vi "trimspace non-reentrant vs reentrant vs inline vs no-subvi.vi"() -> ()   [LabVIEW 2020]
panel:
  out "inside 4":i32
  out "[\\t\\n\\r\\s] 3":string
  out "outside 4":i32
  out "inside 3":i32
  out "[\\t\\n\\r\\s] 2":string
  out "outside 3":i32
  out "[\\t\\n\\r\\s]":string
  out "[\\t\\s]":string
  out "inside 2":i32
  out "outside 2":i32
  out "inside":i32
  out "outside":i32
  out "unit (ms)":dbl[][](graph)
  # "non-reentrant"
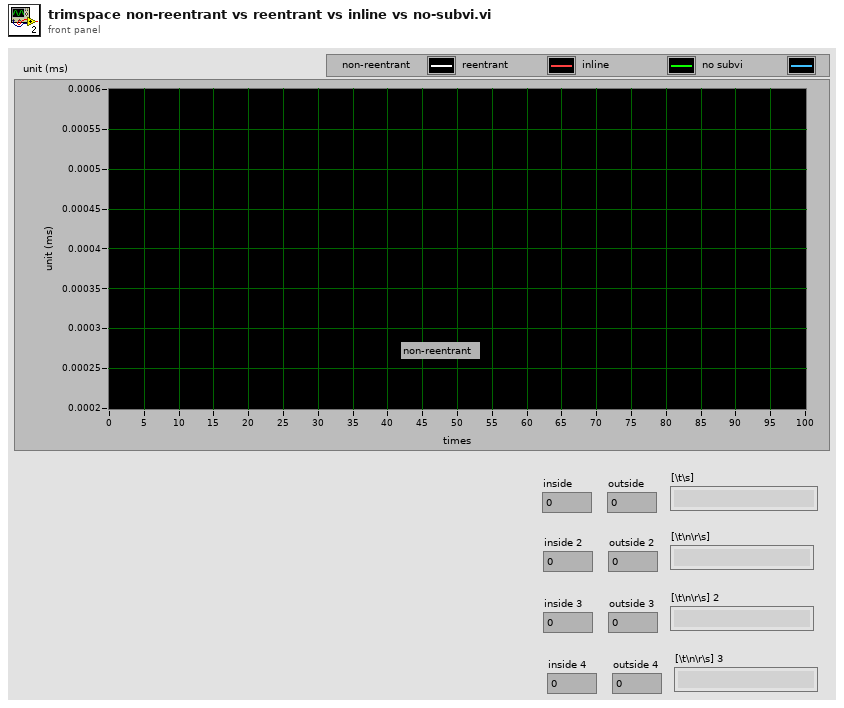
[diagram p1: front panel]
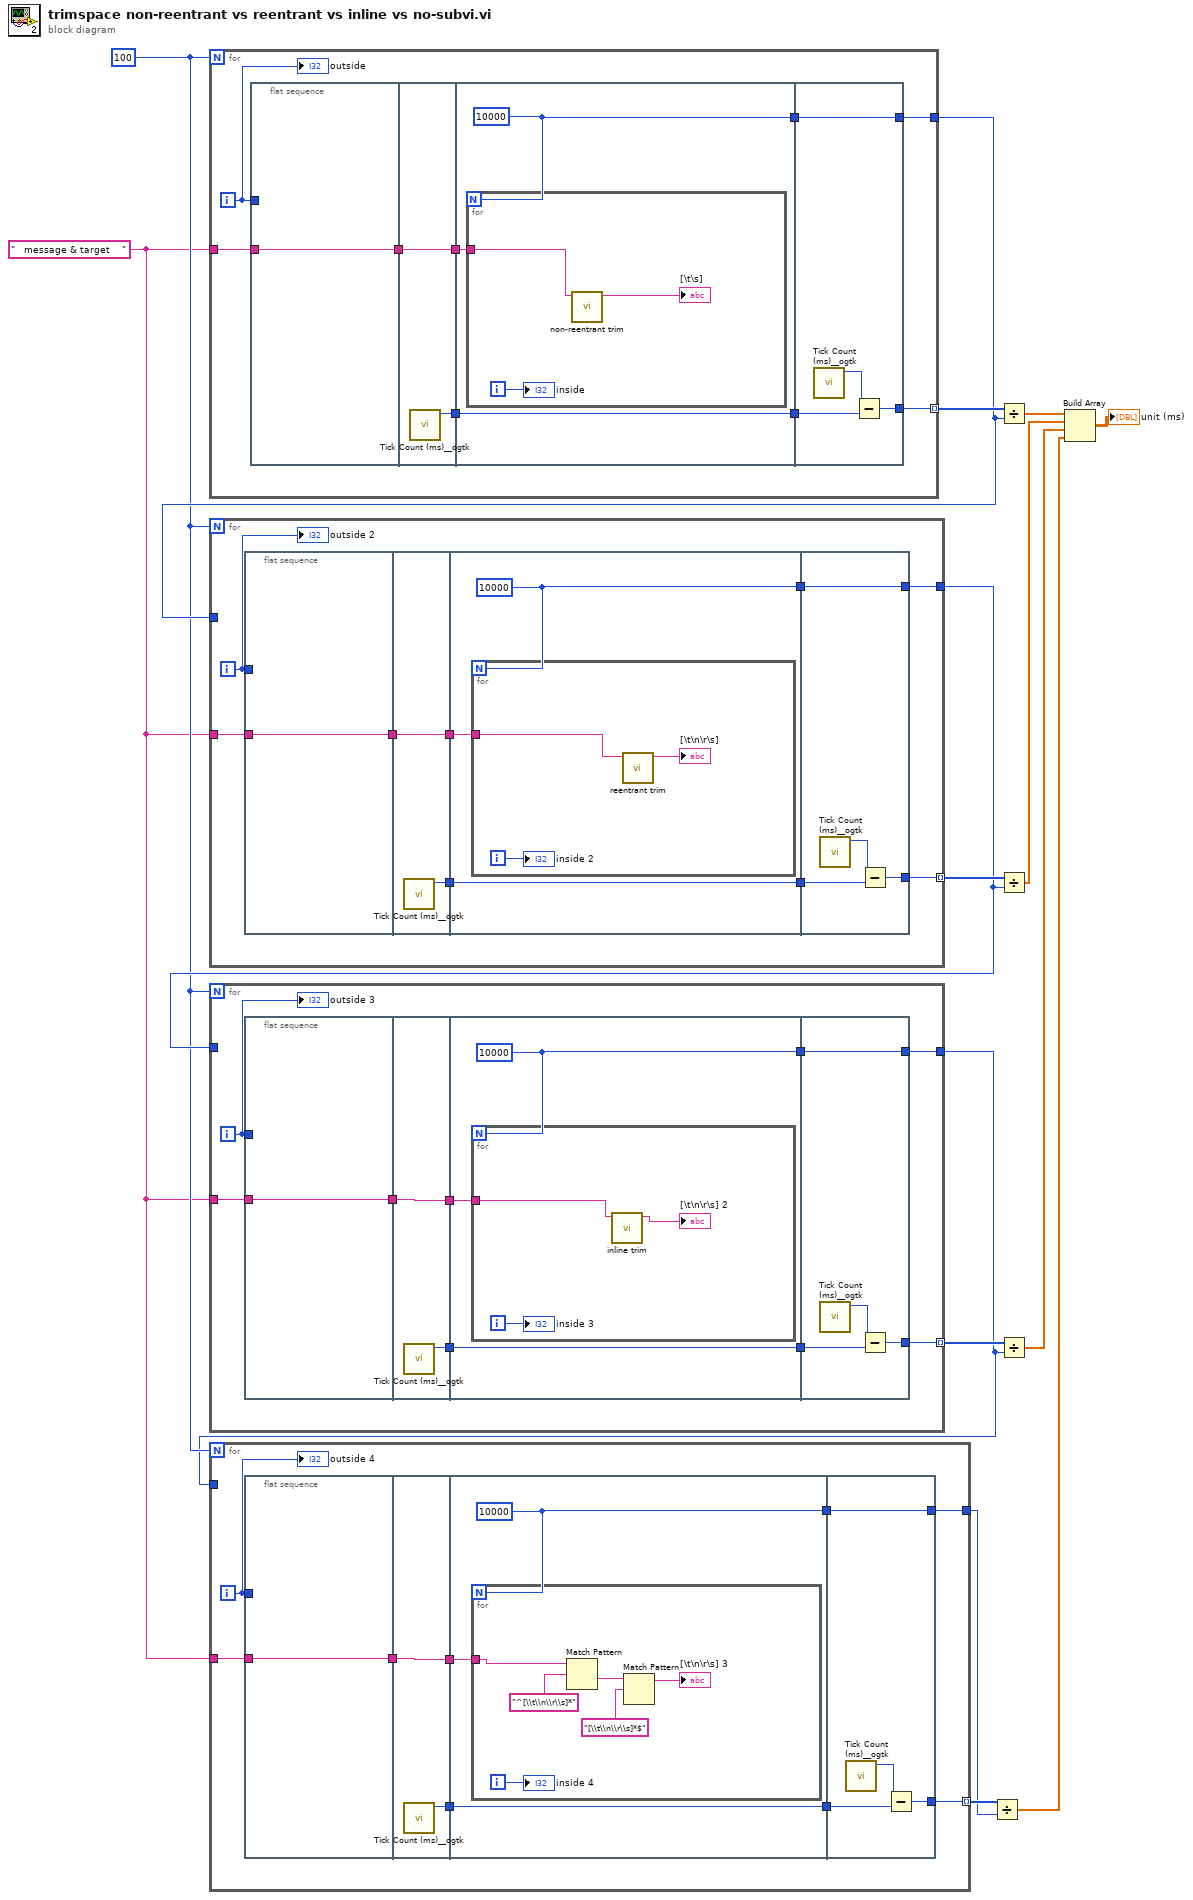
[diagram p0: block diagram]
diagram:
  w4 = "   message & target    " ("string")
  w6 = 100
  n1 = for {
    N: w6 -> [_]
    tunnel: [w22] -> w15 mode=indexing
    tunnel: [w21] -> w12
    tunnel: w4 -> [w16]
    i -> [w19]
    n2 = flat-sequence {
      tunnel: w19 -> [_]
      tunnel: [w25] -> w17
      tunnel: w16 -> [w25]
      tunnel: [w27] -> w24
      tunnel: [w26] -> w18
      tunnel: w17 -> [w26]
      tunnel: w24 -> [w30]
      tunnel: [w30] -> w23
      tunnel: [w29] -> w20
      tunnel: w18 -> [w28]
      tunnel: w23 -> [w36]
      tunnel: [w35] -> w22
      tunnel: [w34] -> w21
      tunnel: w20 -> [w34]
      frame #0 {
      }
      frame #1 {
        n3 = call <userlib>:"Tick Count (ms)__ogtk.vi"() -> ("millisecond timer value"=w27:u32)  [unwired: 10 in, 1 out]
      }
      frame #2 {
        w29 = 10000
        n4 = for {
          N: w29 -> [_]
          tunnel: w28 -> [w32]
          i -> [w33]
          n5 = call "non-reentrant trim.vi"("string in"=w32) -> ("string out"=→"[\\t\\s]":string)  [unwired: 10 in]
          "inside" <- w33
        }
      }
      frame #3 {
        n6 = call <userlib>:"Tick Count (ms)__ogtk.vi"() -> ("millisecond timer value"=w37:u32)  [unwired: 10 in, 1 out]
        n7 = Subtract(x=w37, y=w36) -> (x-y=w35:u32)
      }
    }
    "outside" <- w19
  }
  n8 = for {
    N: w6 -> [_]
    tunnel: [w44] -> w13 mode=indexing
    tunnel: [w43] -> w8
    tunnel: w12 -> [_]
    tunnel: w4 -> [w38]
    i -> [w41]
    n9 = flat-sequence {
      tunnel: w41 -> [_]
      tunnel: [w47] -> w39
      tunnel: w38 -> [w47]
      tunnel: [w49] -> w46
      tunnel: [w48] -> w40
      tunnel: w39 -> [w48]
      tunnel: w46 -> [w52]
      tunnel: [w52] -> w45
      tunnel: [w51] -> w42
      tunnel: w40 -> [w50]
      tunnel: w45 -> [w58]
      tunnel: [w57] -> w44
      tunnel: [w56] -> w43
      tunnel: w42 -> [w56]
      frame #0 {
      }
      frame #1 {
        n10 = call <userlib>:"Tick Count (ms)__ogtk.vi"() -> ("millisecond timer value"=w49:u32)  [unwired: 10 in, 1 out]
      }
      frame #2 {
        w51 = 10000
        n11 = for {
          N: w51 -> [_]
          tunnel: w50 -> [w53]
          i -> [w55]
          n12 = call "reentrant trim.vi"("string in"=w53) -> ("string out"=→"[\\t\\n\\r\\s]":string)  [unwired: 10 in]
          "inside 2" <- w55
        }
      }
      frame #3 {
        n13 = call <userlib>:"Tick Count (ms)__ogtk.vi"() -> ("millisecond timer value"=w59:u32)  [unwired: 10 in, 1 out]
        n14 = Subtract(x=w59, y=w58) -> (x-y=w57:u32)
      }
    }
    "outside 2" <- w41
  }
  n15 = for {
    N: w6 -> [_]
    tunnel: [w66] -> w9 mode=indexing
    tunnel: [w65] -> w5
    tunnel: w4 -> [w60]
    tunnel: w8 -> [_]
    i -> [w63]
    n16 = flat-sequence {
      tunnel: w63 -> [_]
      tunnel: [w69] -> w61
      tunnel: w60 -> [w69]
      tunnel: [w71] -> w68
      tunnel: [w70] -> w62
      tunnel: w61 -> [w70]
      tunnel: w68 -> [w74]
      tunnel: [w74] -> w67
      tunnel: [w73] -> w64
      tunnel: w62 -> [w72]
      tunnel: w67 -> [w80]
      tunnel: [w79] -> w66
      tunnel: [w78] -> w65
      tunnel: w64 -> [w78]
      frame #0 {
      }
      frame #1 {
        n17 = call <userlib>:"Tick Count (ms)__ogtk.vi"() -> ("millisecond timer value"=w71:u32)  [unwired: 10 in, 1 out]
      }
      frame #2 {
        w73 = 10000
        n18 = for {
          N: w73 -> [_]
          tunnel: w72 -> [w75]
          i -> [w77]
          n19 = call "inline trim.vi"("string in"=w75) -> ("string out"=→"[\\t\\n\\r\\s] 2":string)  [unwired: 10 in]
          "inside 3" <- w77
        }
      }
      frame #3 {
        n20 = call <userlib>:"Tick Count (ms)__ogtk.vi"() -> ("millisecond timer value"=w81:u32)  [unwired: 10 in, 1 out]
        n21 = Subtract(x=w81, y=w80) -> (x-y=w79:u32)
      }
    }
    "outside 3" <- w63
  }
  n22 = for {
    N: w6 -> [_]
    tunnel: [w88] -> w3 mode=indexing
    tunnel: [w87] -> w2
    tunnel: w4 -> [w82]
    tunnel: w5 -> [_]
    i -> [w85]
    n23 = flat-sequence {
      tunnel: w85 -> [_]
      tunnel: [w91] -> w83
      tunnel: w82 -> [w91]
      tunnel: [w93] -> w90
      tunnel: [w92] -> w84
      tunnel: w83 -> [w92]
      tunnel: w90 -> [w96]
      tunnel: [w96] -> w89
      tunnel: [w95] -> w86
      tunnel: w84 -> [w94]
      tunnel: w89 -> [w105]
      tunnel: [w104] -> w88
      tunnel: [w103] -> w87
      tunnel: w86 -> [w103]
      frame #0 {
      }
      frame #1 {
        n24 = call <userlib>:"Tick Count (ms)__ogtk.vi"() -> ("millisecond timer value"=w93:u32)  [unwired: 10 in, 1 out]
      }
      frame #2 {
        w95 = 10000
        n25 = for {
          N: w95 -> [_]
          tunnel: w94 -> [w100]
          i -> [w102]
          n26 = Match Pattern(string=w100, regular expression="^[\\t\\n\\r\\s]*") -> (after substring=w97:string)  [unwired: 1 in, 3 out]
          n27 = Match Pattern(string=w97, regular expression="[\\t\\n\\r\\s]*$") -> (before substring=→"[\\t\\n\\r\\s] 3":string)  [unwired: 1 in, 3 out]
          "inside 4" <- w102
        }
      }
      frame #3 {
        n28 = call <userlib>:"Tick Count (ms)__ogtk.vi"() -> ("millisecond timer value"=w106:u32)  [unwired: 10 in, 1 out]
        n29 = Subtract(x=w106, y=w105) -> (x-y=w104:u32)
      }
    }
    "outside 4" <- w85
  }
  n30 = Divide(x=w3, y=w2) -> (x/y=w1:dbl[])
  n31 = Divide(x=w15, y=w12) -> (x/y=w10:dbl[])
  n32 = Divide(x=w13, y=w8) -> (x/y=w11:dbl[])
  n33 = Divide(x=w9, y=w5) -> (x/y=w7:dbl[])
  n34 = Build Array(w10, w11, w7, w1) -> (→"unit (ms)":dbl[][])
